vi "Router - Latency Bmk - Serial CVT FGV - Interelaved Ch.vi"() -> ()   [LabVIEW 2016]
uses:
  <vilib>/Utility/error.llb/DialogType.ctl
  <vilib>/NI/Current Value Table/Type Defs/File Format.ctl
  <vilib>/NI/Current Value Table/Type Defs/Single Tag.ctl
  <vilib>/NI/Current Value Table/Type Defs/Data Types.ctl
  <vilib>/NI/Current Value Table/Type Defs/Tag Grouping set.ctl
  <vilib>/pximc/Initialize Reader Session (DBL).vi
  <vilib>/pximc/Initialize Writer Session (DBL).vi
  <vilib>/pximc/Connect (DBL).vi
  <vilib>/pximc/Acquire Read Region (DBL).vi
  <vilib>/pximc/Acquire Write Region (DBL).vi
  <vilib>/pximc/nipximc.lvlib
  <vilib>/NI/Current Value Table/Current Value Table.lvlib
panel:
  out "Waveform Chart 6":dbl(graph)
  out "Waveform Chart 5":dbl(graph)
  out "Waveform Chart 4":dbl(graph)
  out "Waveform Chart 3":dbl(graph)
  out "Waveform Chart 2":T1(graph)
  out "Waveform Chart":T1(graph)
  out "Array 2":string[](array[string])
  out "Array":string[](array[string])
  in  "Stop Button":bool
  in  "Node 2 Writer Interface":tag="PXI1Slot2" caption="interface"
  in  "Node 2 Writer Connection ID":u16=4
  in  "Node 2 Reader Interface":tag="PXI1Slot2" caption="interface"
  in  "Node 2 Reader Connection ID":u16=3
  in  "Node 1 Writer Interface":tag="PXI1Slot2" caption="interface"
  in  "Node 1 Writer Connection ID":u16=2
  in  "Node 1 Reader Interface":tag="PXI1Slot2" caption="interface"
  in  "Buffer Size":u64=250000 caption="buffer size"
  in  "Connection Timeout (s)":dbl=60.0 caption="timeout in seconds (-1)"
  in  "Node 1 Reader Connection ID":u16=1
  # "Node 1"
  # "Node 2"
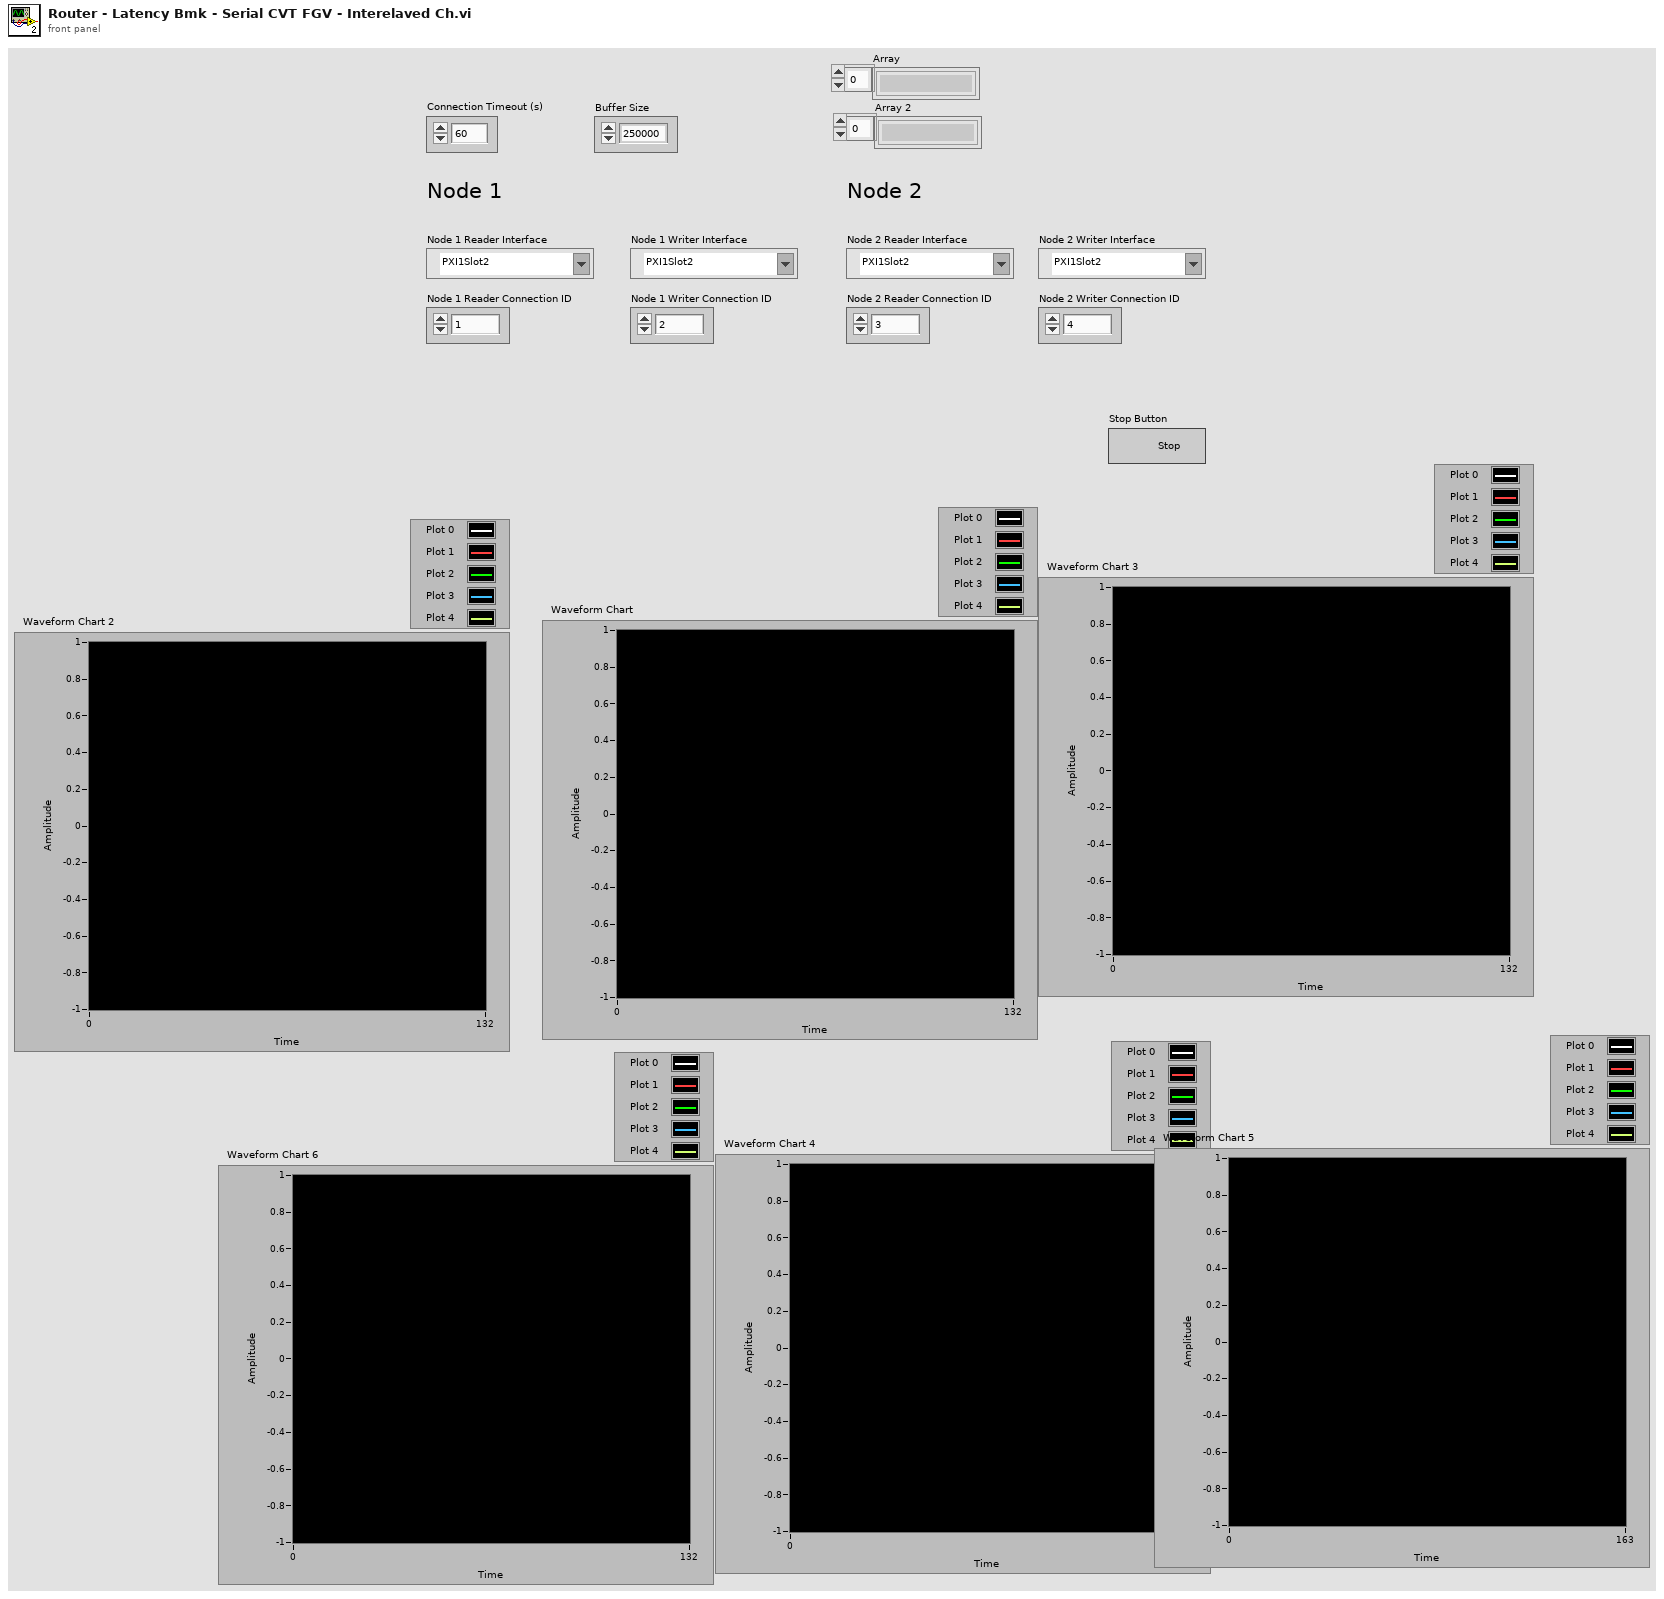
[diagram p1: front panel]
types:
  T1 = cluster{"[0]":dbl, "[1]":dbl, "[2]":dbl, "[3]":dbl, "[4]":dbl, "[5]":dbl, "[6]":dbl, "[7]":dbl, "[8]":dbl}
  T2 = typedef "Current Value Table.lvlib/File Format.ctl" = cluster{"Tags":T3[], "Group Listings":T5[]}
  T3 = typedef "Current Value Table.lvlib/Single Tag.ctl" = cluster{"Data Type":T4, "Name":string, "Value":string, "Description":string}
  T4 = typedef "Current Value Table.lvlib/Data Types.ctl" = enum16{"Double", "Single", "I64", "I32", "I16", "I8", "U64", "U32", "U16", "U8", "String", "Boolean", "Array of U8", "Array of U16", "Array of U32", "Array of U64", "Array of I64", "Array of I32", "Array of I16", "Array of I8", "Array of Double", "Array of Single", "Array of Boolean", "Array of String"}
  T5 = typedef "Current Value Table.lvlib/Tag Grouping set.ctl" = cluster{"Group":string, "Tag Names":string[]}
  T6 = typedef "DialogType.ctl" = u16
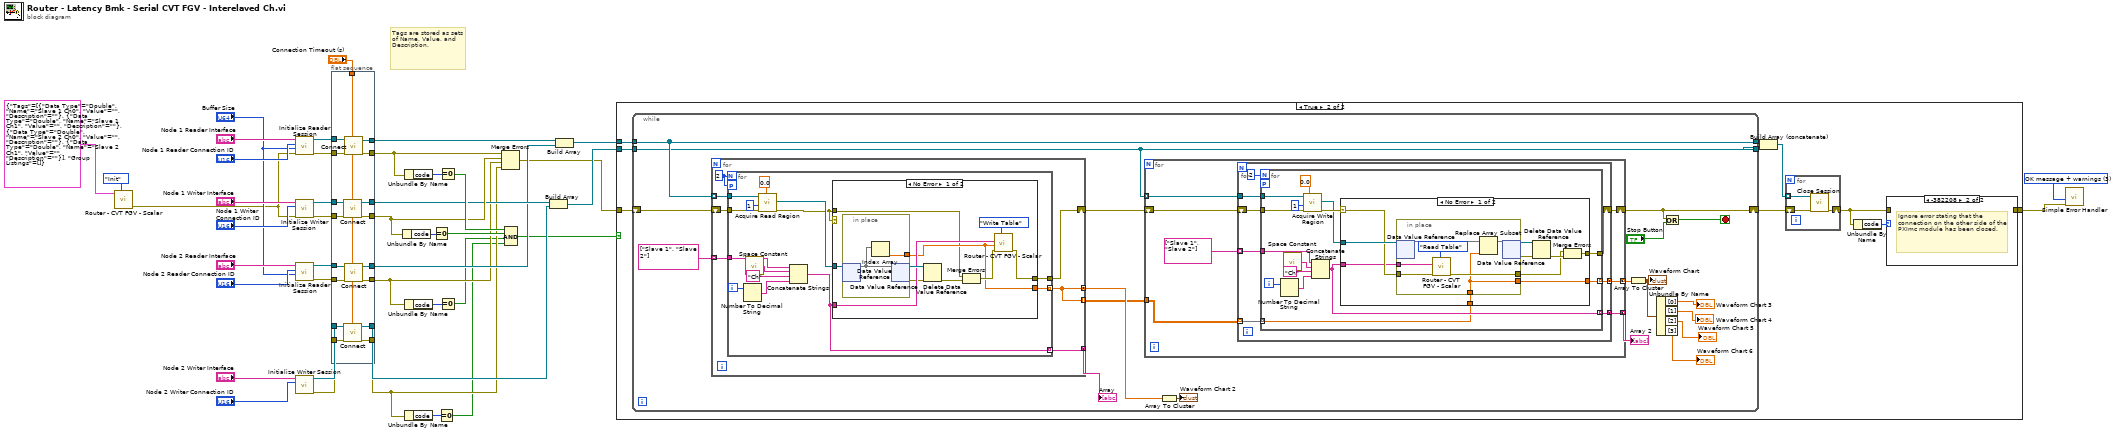
[diagram p0: block diagram]
diagram:
  w38 = T6 3 items=["no dialog", "OK message", "continue or stop message", "OK message + warnings", "continue/stop + warnings"] ("type of dialog (OK msg:1)")
  # "Tags are stored as sets of Name, Value, and Description."
  n1 = call "Router - CVT FGV - Scalar.vi"("FGV Command"=enum16{"Init", "Write Table", "Read Table"}."Init", "CVT Tags to Create"=T2 {"Tags"=[{"Data Type"=enum."Double", "Name"="Slave 1 Ch0", "Value"="", "Description"=""}, {"Data Type"=enum."Double", "Name"="Slave 1 Ch1", "Value"="", "Description"=""}, {"Data Type"=enum."Double", "Name"="Slave 2 Ch0", "Value"="", "Description"=""}, {"Data Type"=enum."Double", "Name"="Slave 2 Ch1", "Value"="", "Description"=""}], "Group Listings"=[]}) -> ("error out"=w7:errorcluster)  [unwired: 8 in, 1 out]
  n2 = call-poly <vilib>:"Initialize Writer Session.vi"("error in (no error)"=w7, "connection id (1)"="Node 1 Writer Connection ID", "interface"="Node 1 Writer Interface") -> ("error out"=w36:errorcluster, "session out"=w35:refnum<k21>)  [unwired: 7 in]
  n3 = call-poly <vilib>:"Initialize Writer Session.vi"("connection id (1)"="Node 2 Writer Connection ID", "interface"="Node 2 Writer Interface") -> ("error out"=w24:errorcluster, "session out"=w25:refnum<k21>)  [unwired: 8 in]
  n4 = call-poly <vilib>:"Initialize Reader Session.vi"("error in (no error)"=w7, "buffer size"="Buffer Size", "writer's connection id (1)"="Node 1 Reader Connection ID", "interface"="Node 1 Reader Interface") -> ("error out"=w41:errorcluster, "session out"=w42:refnum<k21>)  [unwired: 6 in]
  n5 = call-poly <vilib>:"Initialize Reader Session.vi"("buffer size"="Buffer Size", "writer's connection id (1)"="Node 2 Reader Connection ID", "interface"="Node 2 Reader Interface") -> ("error out"=w20:errorcluster, "session out"=w19:refnum<k21>)  [unwired: 7 in]
  n6 = flat-sequence {
    tunnel: w42 -> [w60]
    tunnel: w41 -> [w59]
    tunnel: [w58] -> w15
    tunnel: w36 -> [w57]
    tunnel: w35 -> [w56]
    tunnel: [w55] -> w30
    tunnel: [w54] -> w29
    tunnel: "Connection Timeout (s)" -> [w44]
    tunnel: [w53] -> w16
    tunnel: [w52] -> w13
    tunnel: [w51] -> w11
    tunnel: [w50] -> w12
    tunnel: w25 -> [w49]
    tunnel: w24 -> [w48]
    tunnel: [w47] -> w14
    tunnel: w20 -> [w46]
    tunnel: w19 -> [w45]
    frame #0 {
      n7 = call-poly <vilib>:"Connect.vi"("timeout in seconds (-1)"=w44, "error in (no error)"=w57, "session in"=w56) -> ("error out"=w54:errorcluster, "session out"=w53:refnum<k21>)  [unwired: 7 in]
      n8 = call-poly <vilib>:"Connect.vi"("timeout in seconds (-1)"=w44, "error in (no error)"=w48, "session in"=w49) -> ("error out"=w51:errorcluster, "session out"=w52:refnum<k21>)  [unwired: 7 in]
      n9 = call-poly <vilib>:"Connect.vi"("timeout in seconds (-1)"=w44, "error in (no error)"=w59, "session in"=w60) -> ("error out"=w55:errorcluster, "session out"=w58:refnum<k21>)  [unwired: 7 in]
      n10 = call-poly <vilib>:"Connect.vi"("timeout in seconds (-1)"=w44, "error in (no error)"=w46, "session in"=w45) -> ("error out"=w50:errorcluster, "session out"=w47:refnum<k21>)  [unwired: 7 in]
    }
  }
  n11 = Unbundle By Name(w29) -> ("code"=w33:i32)
  n12 = Unbundle By Name(w30) -> ("code"=w39:i32)
  n13 = Unbundle By Name(w12) -> ("code"=w22:i32)
  n14 = Unbundle By Name(w11) -> ("code"=w27:i32)
  n15 = Equal To 0?(x=w33) -> (x = 0?=w31:bool)
  n16 = Equal To 0?(x=w27) -> (x = 0?=w9:bool)
  n17 = Equal To 0?(x=w39) -> (x = 0?=w32:bool)
  n18 = Equal To 0?(x=w22) -> (x = 0?=w10:bool)
  n19 = Merge Errors(w30, w29, w12, w11) -> (w1:errorcluster)
  n20 = Compound Arithmetic op=AND(w32, w31, w10, w9) -> (w2:bool)
  n21 = Build Array(w16, w13) -> (w4:refnum<k21>[])
  n22 = Build Array(w15, w14) -> (w5:refnum<k21>[])
  n23 = case shown="True" w2 {
    tunnel: w5 -> [_ w71]
    tunnel: w4 -> [_ w70]
    tunnel: [w61 w63] -> w3
    tunnel: w1 -> [w61 w62]
    frame False {
    }
    frame True {
      n24 = while {
        tunnel: w71 -> [w84]
        tunnel: w70 -> [w83]
        shift-right: [w86] -> w68
        shift-left: w62 -> [w85]
        tunnel: [w84] -> w67
        tunnel: [w83] -> w66
        stop <- w88 stop-if-true
        n25 = for {
          tunnel: string[] ["Slave 1", "Slave 2"] -> [w145] mode=indexing
          shift-right: [w144] -> w89
          shift-left: w85 -> [w143]
          tunnel: w84 -> [w142] mode=indexing
          tunnel: [w141] -> w82 mode=concatenating
          tunnel: [w140] -> w78 mode=concatenating
          tunnel: [w140] -> w77 mode=indexing
          w139 = 2
          n26 = for {
            N: w139 -> [_]
            tunnel: w142 -> [w158]
            tunnel: w143 -> [w157]
            tunnel: [w156] -> w144
            tunnel: w145 -> [w150]
            tunnel: [w148] -> w141 mode=indexing
            tunnel: [w147] -> w140 mode=indexing
            workers-P: w139 -> [_]
            i -> [w153]
            n27 = Number To Decimal String(number=w153) -> (decimal integer string=w152:string)  [unwired: 1 in]
            n28 = call <vilib>:"Space Constant.vi"() -> ("String"=w151:string)
            n29 = call-poly <vilib>:"Acquire Read Region.vi"("timeout in seconds (5)"=0.0, "error in (no error)"=w157, "number of elements"=1, "session in"=w158) -> ("error out"=w146:errorcluster, "read region reference"=w159:refnum<data-value>)  [unwired: 4 in, 2 out]
            n30 = Concatenate Strings(w150, w151, "Ch" ("string"), w152) -> (w148:string)
            n31 = case shown="No Error" w146 {
              tunnel: w159 -> [w169 _]
              tunnel: [w163 w172] -> w156
              tunnel: w148 -> [w165 _]
              tunnel: [w161 _] -> w147
              tunnel: w146 -> [w160 w172]
              frame No Error {
                n32 = in-place {
                  in-place-border: [w170] -> w161
                  n33 = in-place-dvr #1(w169) -> (w171:dbl[])  [unwired: 1 out]
                  n34 = Index Array(array=w171) -> (element=w170:dbl)  [unwired: 1 in]
                  n35 = in-place-dvr #1(w171) -> (w168:refnum<data-value>, w162:errorcluster)
                }
                n36 = Delete Data Value Reference(data value reference=w168, error in=w162) -> (error out=w167:errorcluster)  [unwired: 1 out]
                n37 = Merge Errors(w160, w167) -> (w164:errorcluster)
                n38 = call "Router - CVT FGV - Scalar.vi"("FGV Command"=enum16{"Init", "Write Table", "Read Table"}."Write Table", "error in (no error)"=w164, "Tag Write"=w161, "Tag Name"=w165) -> ("error out"=w163:errorcluster)  [unwired: 6 in, 1 out]
              }
              frame Error {
              }
            }
          }
        }
        "Array" <- w82
        n39 = for {
          tunnel: w83 -> [w96] mode=indexing
          shift-right: [w94] -> w86
          shift-left: w89 -> [w95]
          tunnel: [w93] -> w81 mode=concatenating
          tunnel: [w92] -> w80 mode=concatenating
          tunnel: w77 -> [w91]
          n40 = for {
            tunnel: string[] ["Slave 1", "Slave 2"] -> [w105] mode=indexing
            tunnel: w96 -> [w104]
            tunnel: [w100] -> w93 mode=concatenating
            shift-right: [w101] -> w94
            shift-left: w95 -> [w102]
            tunnel: [w99] -> w92 mode=concatenating
            tunnel: w91 -> [w98] mode=indexing
            n41 = for {
              N: 2 -> [_]
              tunnel: w104 -> [w120]
              tunnel: [w118] -> w101
              tunnel: w105 -> [w112]
              tunnel: w102 -> [w111]
              tunnel: [w108] -> w100 mode=indexing
              tunnel: [w107] -> w99 mode=indexing
              tunnel: w98 -> [w106] mode=indexing
              workers-P: _ -> [_]
              i -> [w110]
              n42 = Number To Decimal String(number=w110) -> (decimal integer string=w114:string)  [unwired: 1 in]
              n43 = call <vilib>:"Space Constant.vi"() -> ("String"=w113:string)
              n44 = call-poly <vilib>:"Acquire Write Region.vi"("timeout in seconds (5)"=0.0, "error in (no error)"=w111, "number of elements"=1, "session in"=w120) -> ("error out"=w119:errorcluster, "write region reference"=w117:refnum<data-value>)  [unwired: 4 in, 2 out]
              n45 = Concatenate Strings(w112, w113, "Ch" ("string"), w114) -> (w108:string)
              n46 = case shown="No Error" w119 {
                selector: w119 -> [w126 w138]
                tunnel: w117 -> [w130 _]
                tunnel: [w128 w138] -> w118
                tunnel: w108 -> [w123 _]
                tunnel: [w122 _] -> w107
                tunnel: w106 -> [w121 _]
                frame No Error {
                  n47 = in-place {
                    in-place-border: [w137] -> w124
                    in-place-border: w126 -> [w136]
                    in-place-border: w123 -> [w135]
                    in-place-border: [w131] -> w122
                    in-place-border: w121 -> [w131]
                    n48 = in-place-dvr #2(w130) -> (w133:dbl[])  [unwired: 1 out]
                    n49 = call "Router - CVT FGV - Scalar.vi"("FGV Command"=enum16{"Init", "Write Table", "Read Table"}."Read Table", "error in (no error)"=w136, "Tag Name"=w135) -> ("error out"=w137:errorcluster)  [unwired: 7 in, 1 out]
                    n50 = Replace Array Subset(array=w133, new element=w131) -> (w132:dbl[])  [unwired: 1 in]
                    n51 = in-place-dvr #2(w132) -> (w129:refnum<data-value>, w125:errorcluster)
                  }
                  n52 = Delete Data Value Reference(data value reference=w129, error in=w125) -> (error out=w127:errorcluster)  [unwired: 1 out]
                  n53 = Merge Errors(w124, w127) -> (w128:errorcluster)
                }
                frame Error {
                }
              }
            }
          }
        }
        "Array 2" <- w81
        n54 = Array To Cluster(array=w78) -> (cluster=→"Waveform Chart 2":T1)
        n55 = Array To Cluster(array=w80) -> (cluster=w76:T1)
        "Waveform Chart" <- w76
        n56 = Unbundle By Name(w76) -> ("[0]"=→"Waveform Chart 3":dbl, "[1]"=→"Waveform Chart 4":dbl, "[2]"=→"Waveform Chart 5":dbl, "[3]"=→"Waveform Chart 6":dbl)
        n57 = Or(x=w86, y="Stop Button") -> (x .or. y?=w88:bool)
      }
      n58 = Build Array (concatenate)(w67, w66) -> (w65:refnum<k21>[])
      n59 = for {
        tunnel: w65 -> [w175] mode=indexing
        shift-right: [w173] -> w64
        shift-left: w68 -> [w174]
        n60 = call <vilib>:"Close Session.vi"("error in (no error)"=w174, "session in"=w175) -> ("error out"=w173:errorcluster)  [unwired: 9 in]
      }
      n61 = Unbundle By Name(w64) -> ("code"=w69:i32)
      n62 = case shown="-382208" w69 {
        tunnel: w64 -> [w176 _]
        tunnel: [w176 _] -> w63
        frame 0, Default {
        }
        frame -382208 {
          # "Ignore error stating that the connection on the other side of the PXImc module has been closed."
        }
      }
    }
  }
  n63 = call <vilib>:"Simple Error Handler.vi"("type of dialog (OK msg:1)"=w38, "error in (no error)"=w3) -> ()  [unwired: 3 in, 5 out]
